vi "DHE_TPGetLastValue.vi"(8 "error in (no error)":errorcluster, 9 "swhitches":string[](array[string]), 10 "name":string) -> (0 "error IO":errorcluster, 1 "Limits.InRange":bool, 2 "value":string)   [LabVIEW 2016]
uses:
  DHE_TP_action.ctl
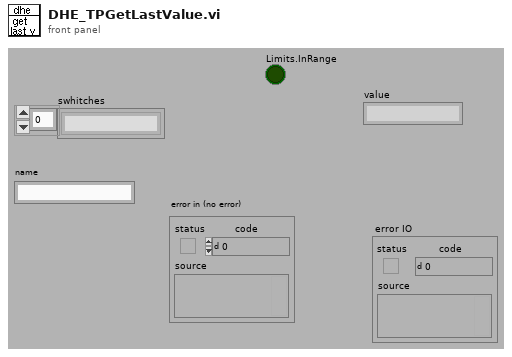
[diagram p1: front panel]
types:
  T1 = typedef "DHE_TP_action.ctl" = enum16{"READ FROM FILE", "GET ALL", "FIND BY NAME", "FIND BY TYPE", "SET VALUE", "CLEAN", "CHANGE", "GET EXPUPDATE"}
  T2 = typedef "DHE_TP.ctl" = cluster{"name":string, "type":string, "R_algor":string[], "board":string, "memory":string, "address":i32, "value":string, "Limits":T3, "unit":string, "params":string, "permissions":string, "W_algor":string[], "description":string, "err_count":i32, "max_err":i32, "read":bool, "lowrej":dbl, "hirej":dbl, "expupd":bool}
  T3 = typedef "DHE_TPLimits.ctl" = cluster{"upper":dbl, "Lower":dbl, "InRange":bool, "nominal":dbl}
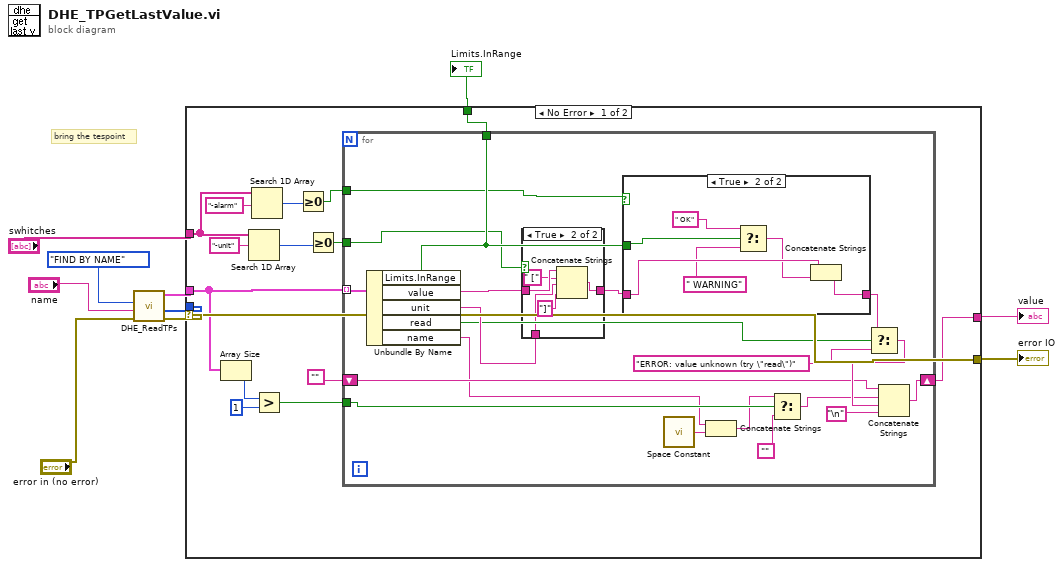
[diagram p0: block diagram]
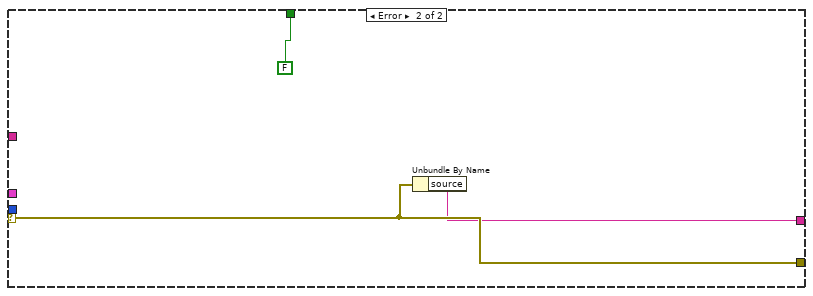
[diagram p4: hidden frame]
diagram:
  # "bring the tespoint"
  n1 = call "DHE_ReadTPs.vi"("error in (no error)"="error in (no error)", "argument"="name", "action"=DHE_TP_action."FIND BY NAME") -> ("error out"=w10:errorcluster, "index"=w8:i32[], "TPs"=w9:T2[])  [unwired: 4 in, 2 out]
  n2 = case shown="No Error" w10 {
    selector: w10 -> [w25 w61]
    tunnel: w9 -> [w14 _]
    tunnel: [w25 w61] -> w5
    tunnel: [w16 w60] -> w3
    tunnel: w8 -> [_ _]
    tunnel: "swhitches" -> [w19 _]
    tunnel: [w24 FALSE ("InRange")] -> w2
    frame No Error {
      n3 = Array Size(array=w14) -> (size(s)=w13:i32)
      n4 = Search 1D Array(1D array=w19, element="-unit") -> (index of element=w20:i32)  [unwired: 1 out]
      n5 = Search 1D Array(1D array=w19, element="-alarm") -> (index of element=w22:i32)  [unwired: 1 out]
      n6 = Greater?(x=w13, y=1) -> (0:w11:bool)
      n7 = Greater Or Equal To 0?(x=w22) -> (x >= 0?=w18:bool)
      n8 = Greater Or Equal To 0?(x=w20) -> (x >= 0?=w17:bool)
      n9 = for {
        tunnel: w14 -> [w38] mode=indexing
        tunnel: [w40] -> w24
        tunnel: w18 -> [w37]
        tunnel: w17 -> [w36]
        shift-right: [w34] -> w16
        shift-left: "" -> [w30]
        tunnel: w11 -> [w32]
        n10 = Unbundle By Name(w38) -> ("Limits.InRange"=w40:bool, "value"=w39:string, "unit"=w44:string, "read"=w41:bool, "name"=w28:string)
        n11 = case shown="True" w36 {
          tunnel: w39 -> [w46 w50]
          tunnel: [w46 w51] -> w45
          tunnel: w44 -> [_ w47]
          frame False {
          }
          frame True {
            n12 = Concatenate Strings(w50, " [" ("string"), w47, "]" ("string")) -> (w51:string)
          }
        }
        n13 = case shown="True" w37 {
          tunnel: w40 -> [_ w56]
          tunnel: w45 -> [w52 w57]
          tunnel: [w52 w58] -> w43
          frame False {
            # "do not send alarm status"
          }
          frame True {
            n14 = Select(t=" OK", s=w56, f=" WARNING") -> (s? t:f=w53:string)
            n15 = Concatenate Strings(w57, w53) -> (w58:string)
          }
        }
        n16 = call <vilib>:"Space Constant.vi"() -> ("String"=w27:string)
        n17 = Concatenate Strings(w28, w27) -> (w26:string)
        n18 = Select(t=w26, s=w32, f="") -> (s? t:f=w29:string)
        n19 = Select(t=w43, s=w41, f="ERROR: value unknown (try \"read\")") -> (s? t:f=w35:string)
        n20 = Concatenate Strings(w30, w29, w35, "\n") -> (w34:string)
      }
    }
    frame Error {
      n21 = Unbundle By Name(w61) -> ("source"=w60:string)
    }
  }
  "error IO" <- w5
  "value" <- w3
  "Limits.InRange" <- w2
